vi "Configure Response - Byte Count.vi"(8 "error in (no error)":errorcluster, 10 "settings":T1 {"Channel Refnum" format="%.0x"; "Linked Channels"."Channel Refnum" format="%.0x"}, 11 "response refnum in":T3 format="%.0x") -> (0 "error out":errorcluster, 3 "response refnum out":T3 format="%.0x")   [LabVIEW 2020, in "Instrument Addon Scripting API.lvlib"]
doc: "Configures the input response with the specified settings.\n \nIf you want to use Linked Channels with the Response Format string, ensure the Channel Refnums used in the Linked Channels parameter already exist before calling this SubVI. \n\nAn error will occur in the following situations: \n- The Response Format string contains duplicate Variable Names. \n- The number of variables in the Response Format string differ from the number of Linked Channels.\n- The Variable Names in the Response Format string differ from the Variable Names used in the Linked Channels parameter."
uses:
  Instrument Addon Scripting API.lvlib
  <vilib>/NI VeriStand/Custom Device API/Custom Device Item Ref.ctl
  TypeDefs/ByteCount Response Settings.ctl
  TypeDefs/Linked Channel.ctl
  Shared Directory/FG Control.ctl
  Shared Directory/Response Parameters.ctl
  Shared Directory/Linked Channel Cluster.ctl
  Shared Directory/Response Wait Type.ctl
  Shared Directory/Constants.vi
  <vilib>/NI VeriStand/Custom Device API/NI VeriStand - Get Item Property.vi
  <vilib>/NI VeriStand/Custom Device API/Get Item Property (String).vi
  <vilib>/NI VeriStand/Custom Device API/Get Item Property (String Array).vi
  <vilib>/NI VeriStand/Custom Device API/Get Item Property (Double).vi
  <vilib>/NI VeriStand/Custom Device API/Get Item Property (U32).vi
  <vilib>/NI VeriStand/Custom Device API/Get Item Property (Boolean).vi
  <vilib>/NI VeriStand/Custom Device API/NI VeriStand - Set Item Property.vi
  <vilib>/NI VeriStand/Custom Device API/Set Item Property (String).vi
  <vilib>/NI VeriStand/Custom Device API/Set Item Property (String Array).vi
  <vilib>/NI VeriStand/Custom Device API/Set Item Property (Double).vi
  <vilib>/NI VeriStand/Custom Device API/Set Item Property (U32).vi
  <vilib>/NI VeriStand/Custom Device API/Set Item Property (Boolean).vi
  Shared Directory/Instrument Addon Shared.lvlib
  <vilib>/NI VeriStand/Custom Device API/Custom Device API.lvlib
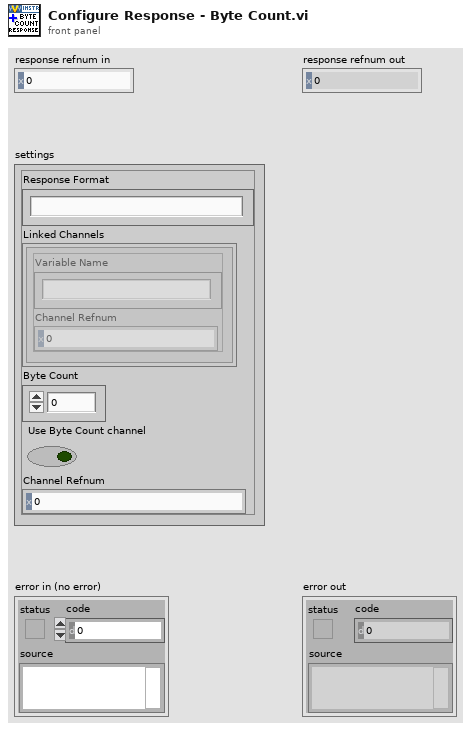
[diagram p1: front panel]
types:
  T1 = typedef "Instrument Addon Scripting API.lvlib/ByteCount Response Settings.ctl" = cluster{"Response Format":string, "Linked Channels":T2[], "Byte Count":i32, "Use Byte Count channel":bool, "Channel Refnum":T3}
  T2 = typedef "Instrument Addon Scripting API.lvlib/Linked Channel.ctl" = cluster{"Variable Name":string, "Channel Refnum":T3}
  T3 = typedef "Custom Device API.lvlib/Custom Device Item Ref.ctl" = u64
  T4 = typedef "Instrument Addon Shared.lvlib/Response Wait Type.ctl" = enum16{"Byte Count", "Wait sec"}
  T5 = typedef "Instrument Addon Shared.lvlib/Response Parameters.ctl" = cluster{"Response":string, "Linked Channels":T6[], "Type Value":dbl, "Wait Type":T4, "Use Channel":bool, "Channel Path":string}
  T6 = typedef "Instrument Addon Shared.lvlib/Linked Channel Cluster.ctl" = cluster{"Variable Name":string, "GUID":string}
  T7 = typedef "Instrument Addon Shared.lvlib/FG Control.ctl" = enum16{"Get", "Set"}
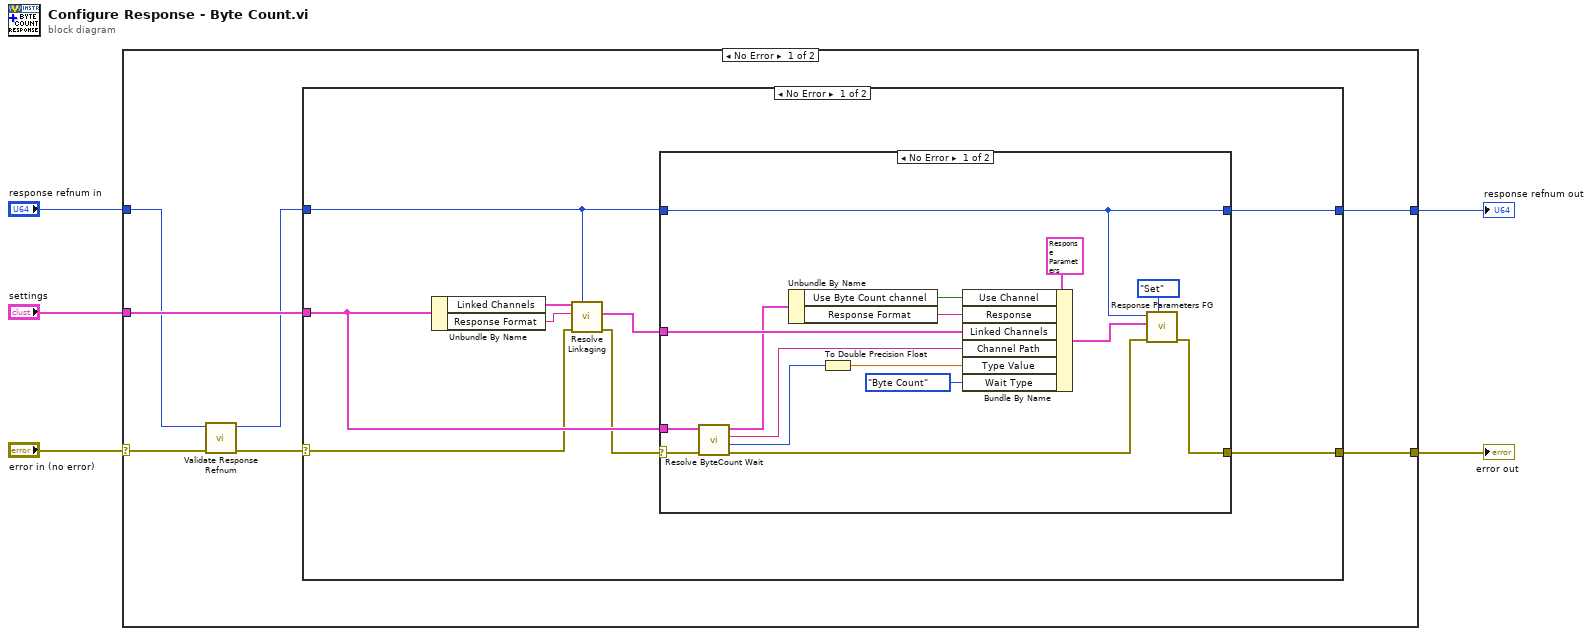
[diagram p0: block diagram]
diagram:
  n1 = case shown="No Error" "error in (no error)" {
    selector: "error in (no error)" -> [w7 w42]
    tunnel: "response refnum in" -> [w9 w43]
    tunnel: "settings" -> [w12 _]
    tunnel: [w11 w43] -> w2
    tunnel: [w10 w42] -> w1
    frame No Error {
      n2 = call "Validate Response Refnum.vi"("error in (no error)"=w7, "response refnum in"=w9) -> ("error out"=w6:errorcluster, "response refnum out"=w8:u64)  [unwired: 8 in]
      n3 = case shown="No Error" w6 {
        selector: w6 -> [w14 w40]
        tunnel: w12 -> [w21 _]
        tunnel: [w20 w41] -> w11
        tunnel: [w19 w40] -> w10
        tunnel: w8 -> [w13 w41]
        frame No Error {
          n4 = Unbundle By Name(w21) -> ("Linked Channels"=w16:T2[], "Response Format"=w15:string)
          n5 = call "Resolve Linkaging.vi"("Command/Response Refnum in"=w13, "error in (no error)"=w14, "Command/Response Format"=w15, "Linked Channels"=w16) -> ("error out"=w18:errorcluster, "Linked Channels out"=w17:T6[])  [unwired: 6 in]
          n6 = case shown="No Error" w18 {
            selector: w18 -> [w27 w38]
            tunnel: w17 -> [w33 _]
            tunnel: [w32 w38] -> w19
            tunnel: w13 -> [w22 w39]
            tunnel: [w22 w39] -> w20
            tunnel: w21 -> [w28 _]
            frame No Error {
              n7 = call "Resolve ByteCount Wait.vi"("error in (no error)"=w27, "Settings in"=w28) -> ("error out"=w26:errorcluster, "Byte Count"=w25:i32, "Channel Path"=w24:string, "Settings out"=w23:T1)  [unwired: 6 in]
              n8 = Unbundle By Name(w23) -> ("Use Byte Count channel"=w29:bool, "Response Format"=w35:string)
              n9 = To Double Precision Float(number=w25) -> (double precision float=w31:dbl)
              n10 = Bundle By Name(cluster=T5 {"Response"="", "Linked Channels"=[], "Type Value"=1.0, "Wait Type"=enum."Wait sec", "Use Channel"=FALSE, "Channel Path"=""} ("Reponse Parameters"), "Use Channel"=w29, "Response"=w35, "Linked Channels"=w33, "Channel Path"=w24, "Type Value"=w31, "Wait Type"=Response_Wait_Type."Byte Count") -> (w34:T5)
              n11 = call "Response Parameters FG.vi"("Action"=FG_Control."Set", "error in (no error)"=w26, "Reponse Parameters"=w34, "Item Ref in"=w22) -> ("error out"=w32:errorcluster)  [unwired: 5 in, 2 out]
            }
            frame Error {
            }
          }
        }
        frame Error {
        }
      }
    }
    frame Error {
    }
  }
  "error out" <- w1
  "response refnum out" <- w2
